vi "SSC DAQmx Timing.vi"(0 "DAQmx SSC in":T1[](array[typedef]), 1 "Sample Mode":i32(ring)=10123 items=["Finite Samples"=10178, "Continuous Samples"=10123, "Hardware Timed Single Point"=12522], 2 "Samples":i32=1000, 5 "Sample Rate":dbl=1000.0 format="%0.2f", 7 "Source":tag="OnboardClock", 9 "Active Edge":i32(ring)=10280 items=["Rising"=10280, "Falling"=10171], 11 "error in":errorcluster, 12 "Set Reference Clock Source?":bool, 13 "RefClk.Src":tag="PXIe_Clk100") -> (4 "DAQmx SSC out":T1[](array[typedef]), 15 "error out":errorcluster)   [LabVIEW 2020]
doc: "Sets the source of the Sample Clock, the rate of the Sample Clock, and the number of samples to acquire or generate.\nOptionally set the reference clock source."
uses:
  Pin Map/SSC DAQmx.ctl
  <vilib>/DAQmx/configure/timing.llb/DAQmx Timing (Sample Clock).vi
  <resource>/objmgr/daqmx.rc
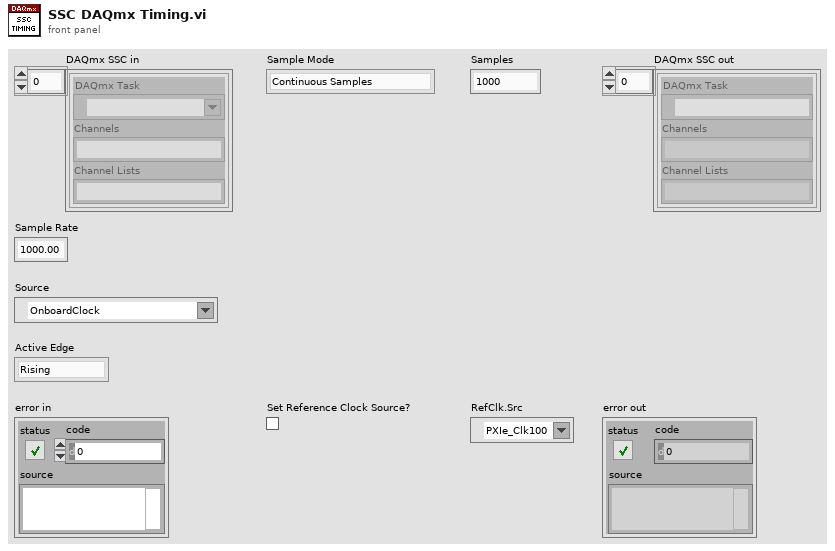
[diagram p1: front panel]
types:
  T1 = typedef "SSC DAQmx.ctl" = cluster{"DAQmx Task ":refnum<k21>, "Channels":string, "Channel Lists":string}
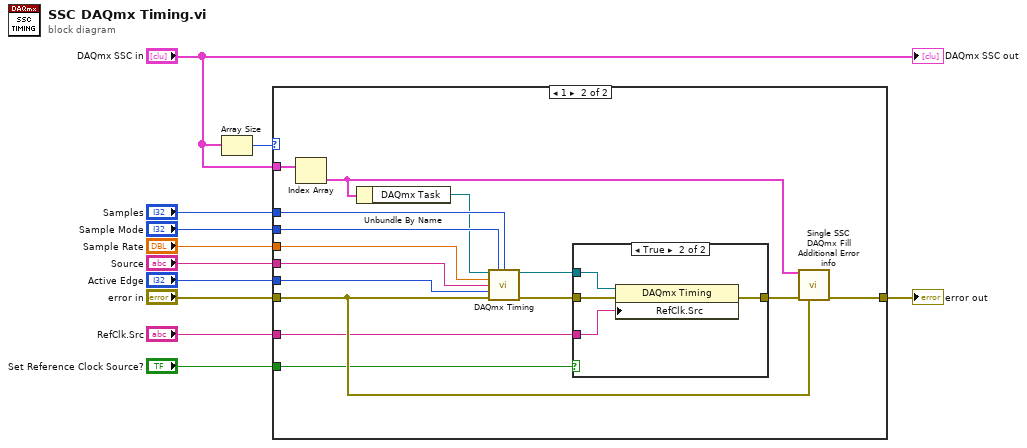
[diagram p0: block diagram]
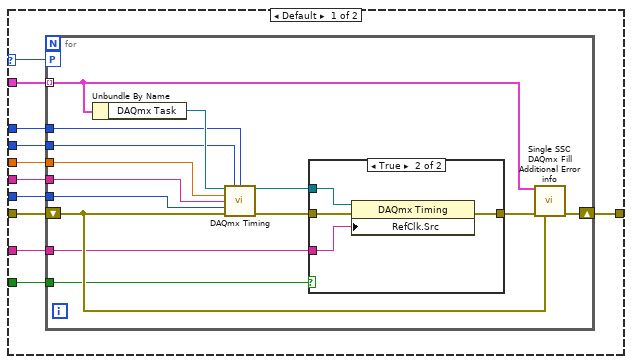
[diagram p2: hidden frame]
diagram:
  n1 = Array Size(array="DAQmx SSC in") -> (size(s)=w9:i32)
  n2 = case shown="1" w9 {
    selector: w9 -> [w20 _]
    tunnel: [w22 w56] -> w11
    tunnel: "error in" -> [w21 w55]
    tunnel: "DAQmx SSC in" -> [w19 w54]
    tunnel: "Samples" -> [w18 w53]
    tunnel: "Sample Mode" -> [w17 w52]
    tunnel: "Sample Rate" -> [w16 w51]
    tunnel: "RefClk.Src" -> [w15 w50]
    tunnel: "Source" -> [w14 w49]
    tunnel: "Active Edge" -> [w13 w48]
    tunnel: "Set Reference Clock Source?" -> [w12 w47]
    frame Default {
      n3 = for {
        tunnel: w19 -> [w35] mode=indexing
        workers-P: w20 -> [_]
        shift-right: [w36] -> w22
        shift-left: w21 -> [w32]
        tunnel: w18 -> [w29]
        tunnel: w17 -> [w28]
        tunnel: w16 -> [w27]
        tunnel: w15 -> [w26]
        tunnel: w14 -> [w25]
        tunnel: w13 -> [w24]
        tunnel: w12 -> [w23]
        n4 = Unbundle By Name(w35) -> ("DAQmx Task"=w30:refnum<k21>)
        n5 = call-poly <vilib>:"DAQmx Timing.vi"("task/channels in"=w30, "sample mode"=w28, "samples per channel"=w29, "rate"=w27, "source"=w25, "active edge"=w24, "error in"=w32) -> ("task out"=w34:refnum<k21>, "error out"=w33:errorcluster)  [unwired: 7 in]
        n6 = case shown="True" w23 {
          tunnel: w34 -> [_ w41]
          tunnel: w33 -> [w37 w40]
          tunnel: [w37 w39] -> w31
          tunnel: w26 -> [_ w38]
          frame False {
          }
          frame True {
            n7 = property class="DAQmx Timing"(reference=w41, error in=w40, "RefClk.Src"=w38) -> (error out=w39:errorcluster)  [unwired: 1 out]
          }
        }
        n8 = call "Single SSC DAQmx Fill Additional Error info.vi"("DAQmx SSC in"=w35, "error in"=w31, "previous error in"=w32) -> ("error out"=w36:errorcluster)  [unwired: 12 in]
      }
    }
    frame 1 {
      n9 = Index Array(array=w54) -> (element=w42:T1)  [unwired: 1 in]
      n10 = Unbundle By Name(w42) -> ("DAQmx Task"=w43:refnum<k21>)
      n11 = call-poly <vilib>:"DAQmx Timing.vi"("task/channels in"=w43, "sample mode"=w52, "samples per channel"=w53, "rate"=w51, "source"=w49, "active edge"=w48, "error in"=w55) -> ("task out"=w46:refnum<k21>, "error out"=w45:errorcluster)  [unwired: 7 in]
      n12 = case shown="True" w47 {
        tunnel: w46 -> [_ w61]
        tunnel: w45 -> [w57 w60]
        tunnel: [w57 w59] -> w44
        tunnel: w50 -> [_ w58]
        frame False {
        }
        frame True {
          n13 = property class="DAQmx Timing"(reference=w61, error in=w60, "RefClk.Src"=w58) -> (error out=w59:errorcluster)  [unwired: 1 out]
        }
      }
      n14 = call "Single SSC DAQmx Fill Additional Error info.vi"("DAQmx SSC in"=w42, "error in"=w44, "previous error in"=w55) -> ("error out"=w56:errorcluster)  [unwired: 12 in]
    }
  }
  "error out" <- w11
  "DAQmx SSC out" <- "DAQmx SSC in"
